vi "ma_resample single-shot (FIR).vi"(4 "Filter parameters":T1 {"half duration" format="%.2f"; "FIR index step" format="%.2f"; "scaled filter" format="%.2p"}, 6 "#elements":i32, 8 "error in":errorcluster, 9 "t0":timestamp format="%<%.4X>T", 10 "dt":dbl=1.0 format="%.2p", 11 "waveform in":waveform(dbl)) -> (0 "error out":errorcluster, 3 "resampled waveform out":waveform(dbl))   [LabVIEW 2020, in "NI_MAPro.lvlib"]
doc: "This VI re-samples an unevenly sampled input signal to an evenly sampled waveform according to specified t0 and dt. If the specified t0 value is less than the first value of input X-array (that is the timestamp of the first input sample), then the VI will coerce t0 to the first valid value (greater than X(0)) that also fulfill the relation:\n\nT0_adjusted - t0_in = n * dt_in\n\nThis guarranty that any later comparison of waveforms will be correct with repsect to absolute time."
uses:
  NI_MAPro.lvlib
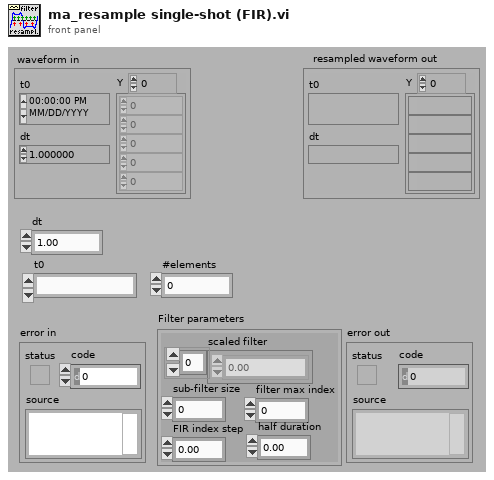
[diagram p1: front panel]
types:
  T1 = cluster{"scaled filter":dbl[], "sub-filter size":i32, "filter max index":i32, "FIR index step":dbl, "half duration":dbl}
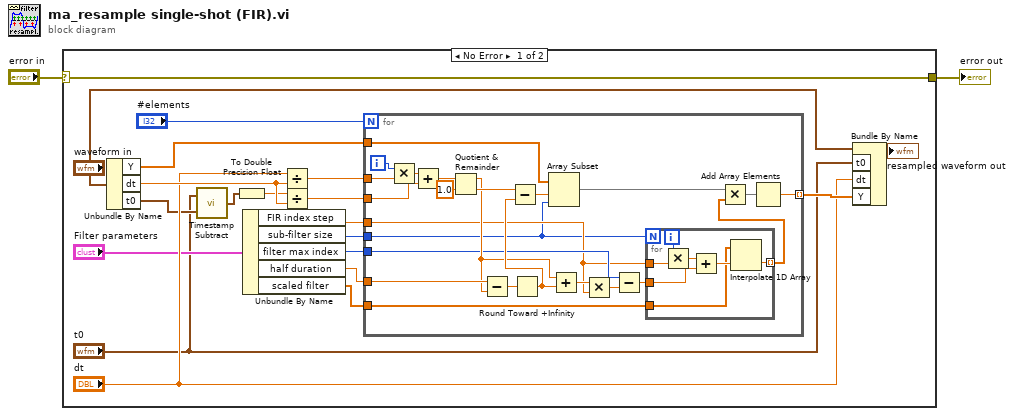
[diagram p0: block diagram]
diagram:
  n1 = case shown="No Error" "error in" {
    selector: "error in" -> [w15 w54]
    tunnel: [w15 w54] -> w1
    frame No Error {
      n2 = Unbundle By Name("waveform in") -> ("Y"=w20:dbl[], "dt"=w14:dbl, "t0"=w6:timestamp)
      n3 = call "Timestamp Subtract.vi"("y"=w6, "x"="t0") -> ("x - y"=w4:timestamp)
      n4 = To Double Precision Float(number=w4) -> (double precision float=w3:dbl)
      n5 = Unbundle By Name("Filter parameters") -> ("FIR index step"=w8:dbl, "sub-filter size"=w9:i32, "filter max index"=w7:i32, "half duration"=w10:dbl, "scaled filter"=w11:dbl[])
      n6 = Divide(x="dt", y=w14) -> (x/y=w18:dbl)
      n7 = Divide(x=w3, y=w14) -> (x/y=w17:dbl)
      n8 = for {
        N: "#elements" -> [_]
        tunnel: w18 -> [w45]
        tunnel: w20 -> [w36]
        tunnel: [w23] -> w19 mode=indexing
        tunnel: w17 -> [w43]
        tunnel: w10 -> [w40]
        tunnel: w9 -> [w25]
        tunnel: w8 -> [w30]
        tunnel: w7 -> [w31]
        tunnel: w11 -> [w28]
        i -> [w46]
        n9 = Multiply(x=w46, y=w45) -> (x*y=w44:dbl)
        n10 = Add(x=w44, y=w43) -> (x+y=w42:dbl)
        n11 = Quotient & Remainder(x=w42, y=1.0) -> (x-y*floor(x/y)=w34:dbl, floor(x/y)=w38:dbl)
        n12 = Subtract(x=w40, y=w34) -> (x-y=w39:dbl)
        n13 = Round Toward +Infinity(x=w39) -> (ceil(x): smallest int >= x=w37:dbl)
        n14 = Subtract(x=w38, y=w37) -> (x-y=w24:dbl)
        n15 = Array Subset(array=w36, index=w24, length=w25) -> (w35:dbl[])
        n16 = Add(x=w34, y=w37) -> (x+y=w33:dbl)
        n17 = Multiply(x=w33, y=w30) -> (x*y=w32:dbl)
        n18 = Subtract(x=w31, y=w32) -> (x-y=w29:dbl)
        n19 = for {
          N: w25 -> [_]
          tunnel: w30 -> [w48]
          tunnel: w29 -> [w52]
          tunnel: w28 -> [w50]
          tunnel: [w49] -> w26 mode=indexing
          i -> [w47]
          n20 = Multiply(x=w47, y=w48) -> (x*y=w53:dbl)
          n21 = Add(x=w53, y=w52) -> (x+y=w51:dbl)
          n22 = Interpolate 1D Array(1:w51, 2:w50) -> (0:w49:dbl)
        }
        n23 = Multiply(x=w35, y=w26) -> (x*y=w27:dbl[])
        n24 = Add Array Elements(numeric array=w27) -> (sum=w23:dbl)
      }
      n25 = Bundle By Name(cluster="waveform in", "t0"="t0", "dt"="dt", "Y"=w19) -> (→"resampled waveform out":waveform(dbl))
    }
    frame Error {
    }
  }
  "error out" <- w1
